vi "Test Controller Verify User.vi"(8 "error in (no error)":errorcluster, 11 "Test Case In":refnum<class "Controller Test.lvclass">) -> (0 "error out":errorcluster, 3 "Test Case Out":refnum<class "Controller Test.lvclass">)   [LabVIEW 2020, in "Controller Test.lvclass"]
uses:
  Controller Test.lvclass
  Controller Test.lvclass/Controller Test.ctl
  01074fa8-ee8a-411d-bc8b-fc92c4f90959.vi
  ATM Controller/ATM Controller.lvclass
  ATM Controller/State.ctl
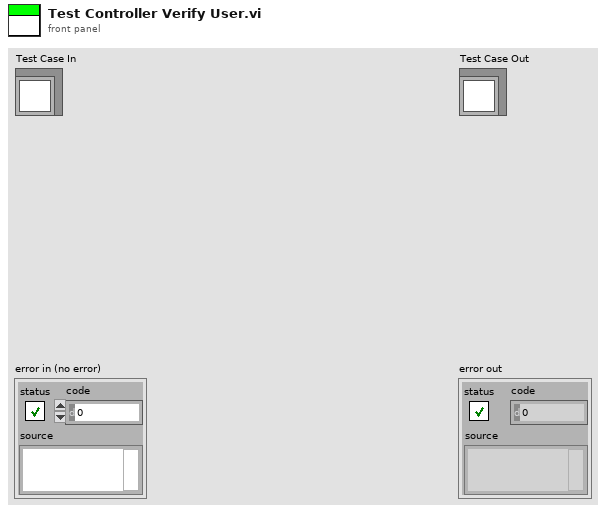
[diagram p1: front panel]
types:
  T1 = typedef "ATM Controller.lvclass/State.ctl" = enum16{"Start", "Card Inserted", "Verification Failed", "Verification Succeeded", "Return Card"}
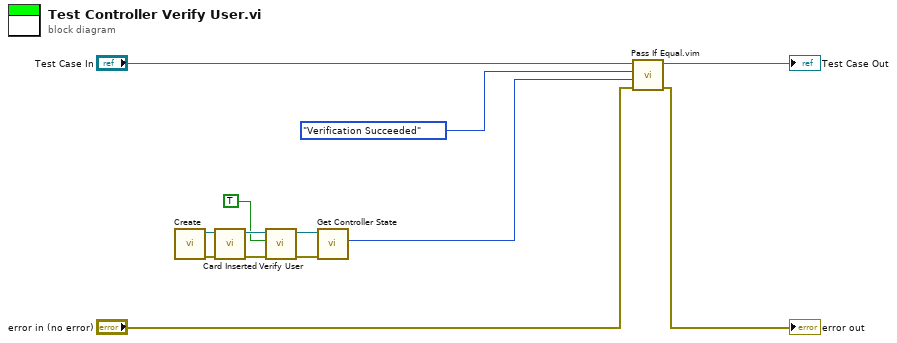
[diagram p0: block diagram]
diagram:
  n1 = call "Create.vi"() -> ("error out"=w9:errorcluster, "ATM Controller out"=w5:refnum<class "ATM Controller.lvclass">)  [unwired: 10 in]
  n2 = call "Card Inserted.vi"("error in (no error)"=w9, "ATM Controller in"=w5) -> ("error out"=w6:errorcluster, "ATM Controller out"=w3:refnum<class "ATM Controller.lvclass">)  [unwired: 8 in]
  n3 = call "Verify User.vi"("error in (no error)"=w6, "Verified?"=TRUE, "ATM Controller in"=w3) -> ("error out"=w4:errorcluster, "ATM Controller out"=w2:refnum<class "ATM Controller.lvclass">)  [unwired: 7 in]
  n4 = call "Get Controller State.vi"("error in (no error)"=w4, "ATM Controller in"=w2) -> ("ATM State"=w8:T1)  [unwired: 7 in, 2 out]
  n5 = call "Pass If Equal.vim"("error in (no error)"="error in (no error)", "Actual"=w8, "Expected"=State."Verification Succeeded" ("ATM State"), "LUnit Test Case In"="Test Case In") -> ("error out"=→"error out":errorcluster, "LUnit Test Case Out"=→"Test Case Out":refnum<class "Controller Test.lvclass">)  [unwired: 6 in]
